vi "acquire-sequence-to-disk-subvi.vi"(0 "Image Size":T7={"H Bin"=1.0, "V Bin"=1.0, "Left"=1.0, "Right"=1024.0, "Top"=1.0, "Bottom"=1024.0} {"V Bin" min=0.0; "H Bin" min=0.0 step=1.0}, 1 "Description Info":string, 2 "Operation":enum16{"Start", "Continue", "Finish"}(ring), 3 "Number of frames to acquire":i32, 5 "Display?":bool, 7 "State In":T1 {"Height" format="%.2f"; "Width" format="%.2f"}, 9 "Frames per acquisition file":u32, 11 "Sequence files handle":T8, 12 "Pressing stop automatically runs finish?":bool=TRUE, 13 "Display Window Title":string="Acquired Image", 14 "Display Window Number":i32) -> (4 "Done?":bool, 6 "State Out":T1 {"Height" format="%.2f"; "Width" format="%.2f"}, 10 "Sequence files handle out":T8, 15 "Error Out":errorcluster)   [LabVIEW 2014]
uses:
  SubVIs/ctt's/Video acquisition state1.ctl
  <vilib>/vision/Image Controls.llb/IMAQ Image.ctl
  Glimpse-master/Glimpse core/Seq file v 1/Offset table.ctl
  Glimpse-master/Glimpse core/Seq file v 1/Offset.ctl
  Glimpse-master/Glimpse core/Seq file v 1/file number.ctl
  Header2 file.ctl
  SubVIs/Initilize Globals.vi
  Stage Control/Stage SubVis/stage-controller-globals.vi
  Shutter Control/Shutter SubVis/Global Shutter Variables - SubVI.vi
  flow-rate-global.vi
  hardware names - global.vi
panel:
  in  "Laser Shutter (to get strings only)":T6(radio)
  out "Frame interval (ms)":i16
  out "TTB element zero":u32
  out "Time of 1st frame":dbl
  out "Frames Acquired":u32(slide) scale=0.0..10000.0
  in  "Stop":bool
  out "Sequence files directory path":path
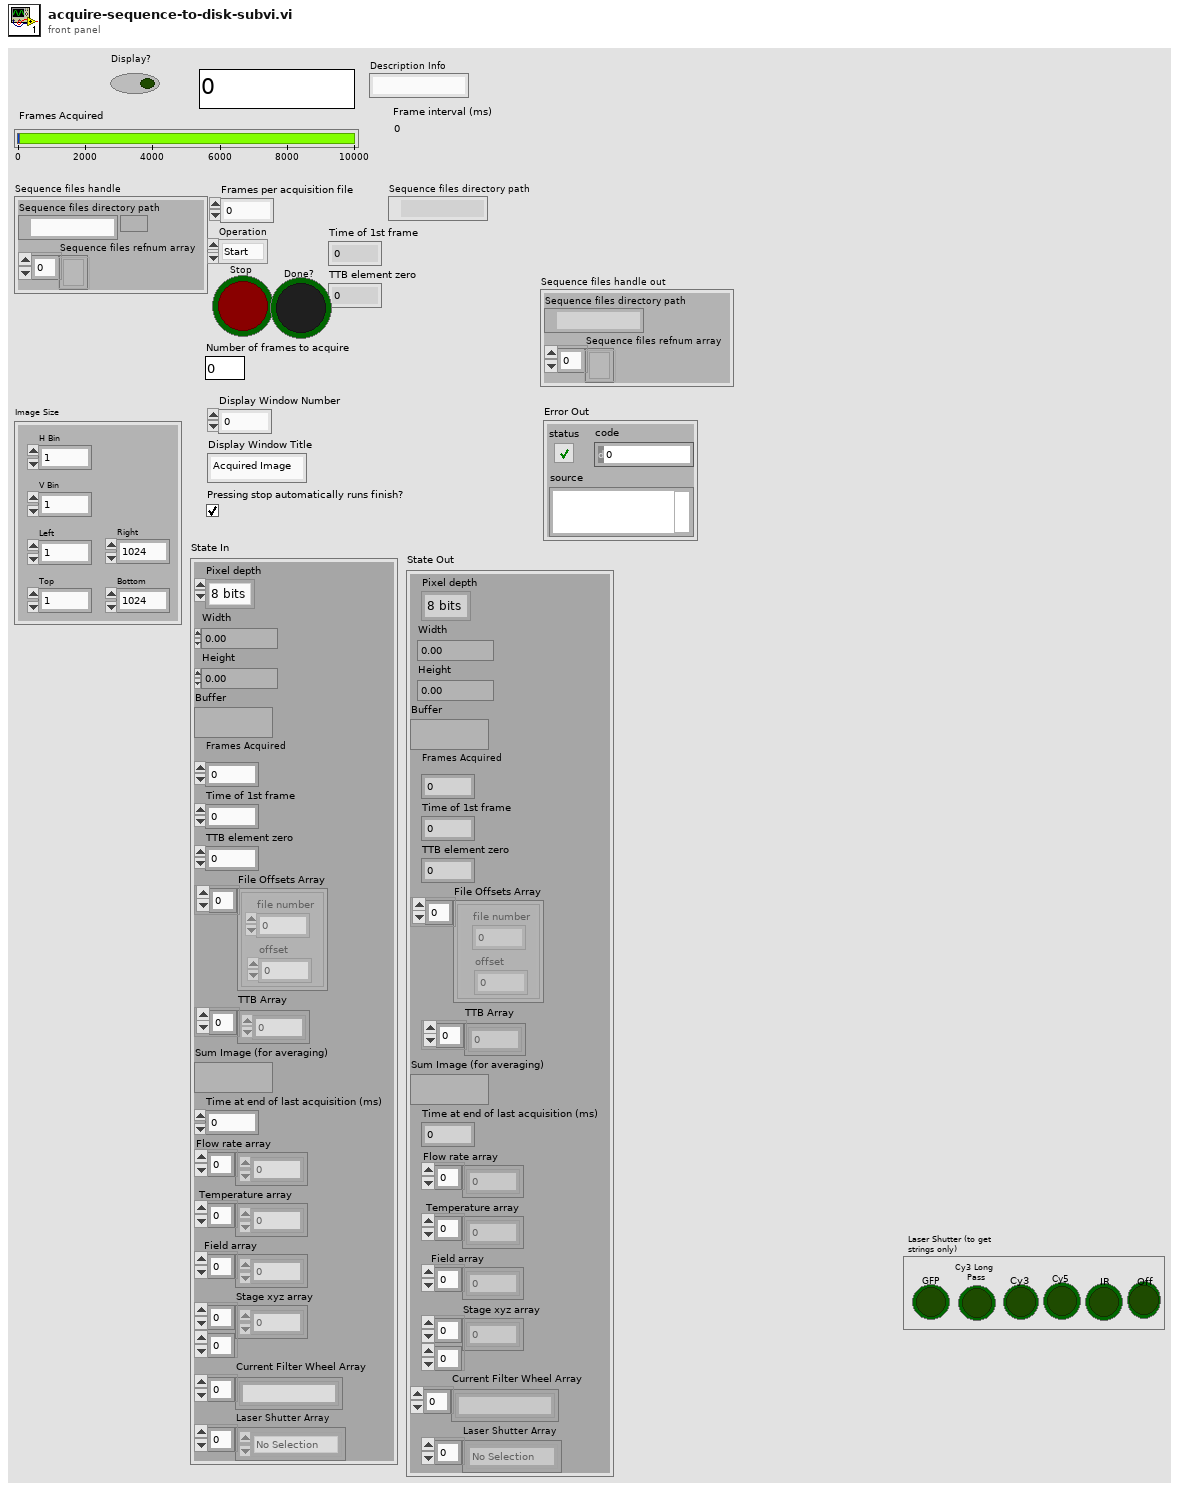
[diagram p1: front panel]
types:
  T1 = typedef "Video acquisition state1.ctl" = cluster{"Pixel depth":enum32{"8 bits", "16 bits", "Float", "Complex", "RGB Chunky", "Compressed"}, "Width":dbl, "Height":dbl, "Buffer":T2, "Frames Acquired":u32, "Time of 1st frame":dbl, "TTB element zero":u32, "File Offsets Array":T3, "TTB Array":u32[], "Sum Image (for averaging)":T2, "Time at end of last acquisition (ms)":u32, "Flow rate array":dbl[], "Temperature array":dbl[], "Field array":u16[], "Stage xyz array":dbl[][], "Current Filter Wheel Array":string[], "Laser Shutter Array":enum32{"No Selection", "GFP", "Cy3 Long \nPass", "Cy3", "Cy5", "Off", "IR"}[]}
  T2 = typedef "IMAQ Image.ctl" = refnum<image>
  T3 = typedef "Offset table.ctl" = cluster{"offset":T4, "file number":T5}[]
  T4 = typedef "Offset.ctl" = i32
  T5 = typedef "file number.ctl" = u8
  T6 = enum32{"No Selection", "GFP", "Cy3 Long \nPass", "Cy3", "Cy5", "Off", "IR"}
  T7 = cluster{"H Bin":dbl, "V Bin":dbl, "Left":dbl, "Right":dbl, "Top":dbl, "Bottom":dbl}
  T8 = cluster{"Sequence files directory path":path, "Sequence files refnum array":refnum<file>[]}
  T9 = enum32{"8 bits", "16 bits", "Float", "Complex", "RGB Chunky", "Compressed"}
  T10 = enum32{"No Selection", "GFP", "Cy3 Long \nPass", "Cy3", "Cy5", "Off", "IR"}[]
  T11 = typedef "Header2 file.ctl" = cluster{"Camera":string, "Microscope":string, "Microscope software version":string, "Flow rate array":dbl[], "Temperature array":dbl[], "Field array":u16[], "Is header2 info present?":bool, "Description Info":string, "Stage xyz array":dbl[][], "Current Filter Wheel Array":string[], "Laser Shutter Array":enum32{"No Selection", "GFP", "Cy3 Long \nPass", "Cy3", "Cy5", "Off", "IR"}[], "Laser Shutter Names":string[]}
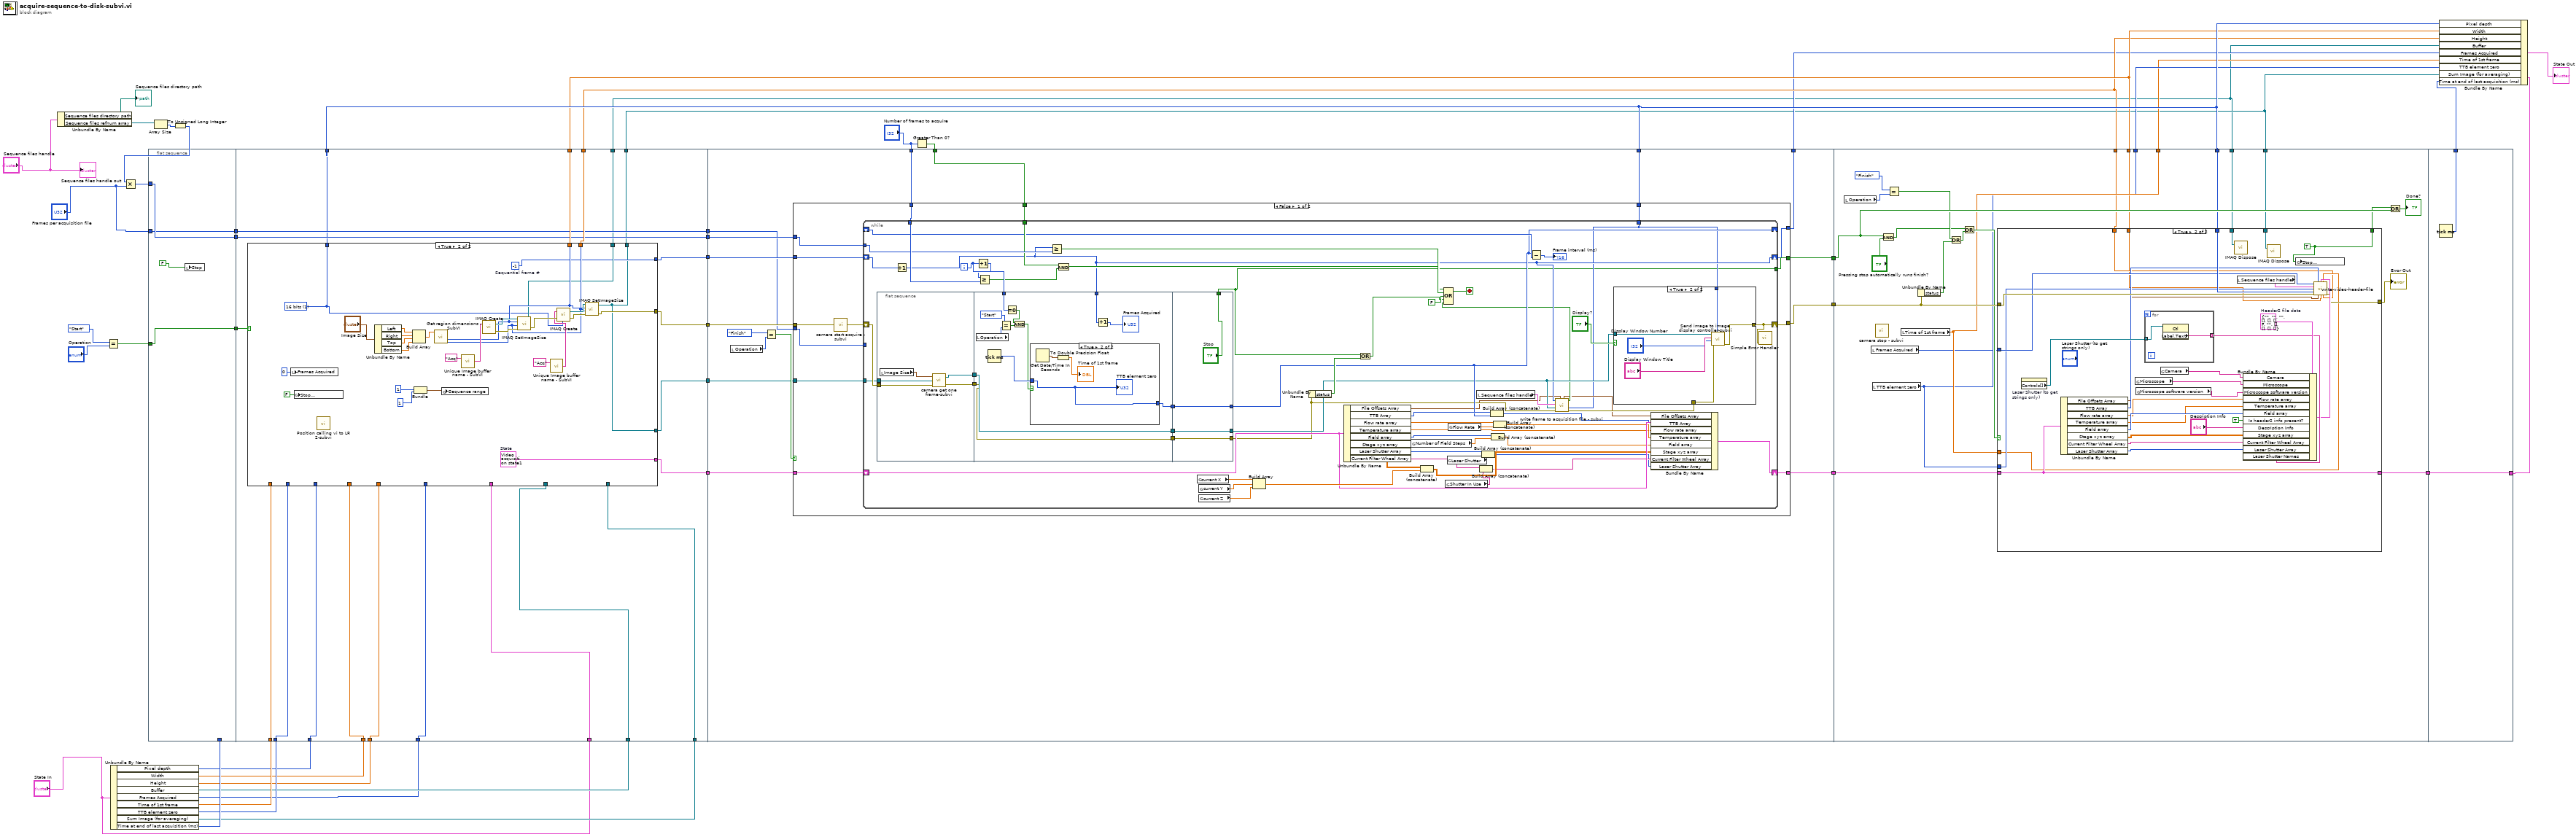
[diagram p0: block diagram]
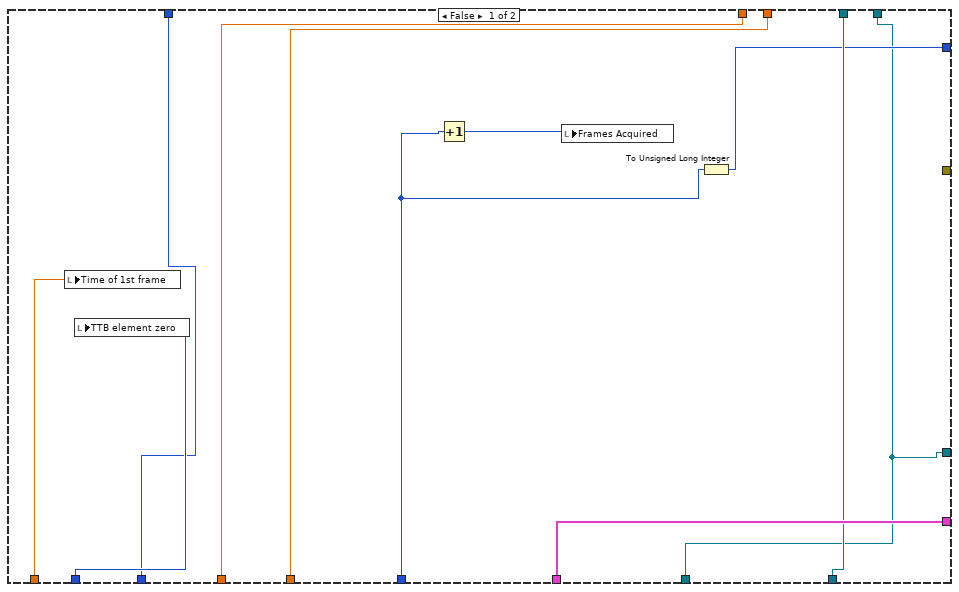
[diagram p2: hidden frame]
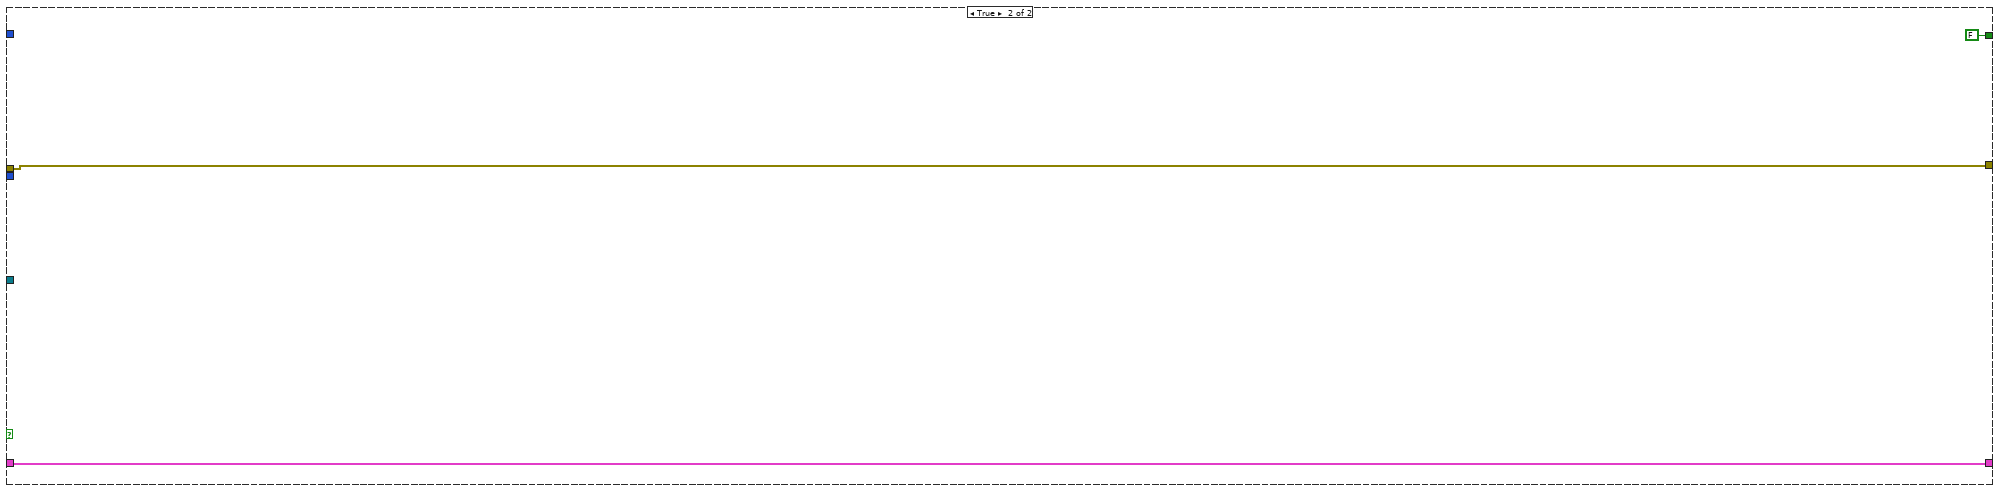
[diagram p5: hidden frame]
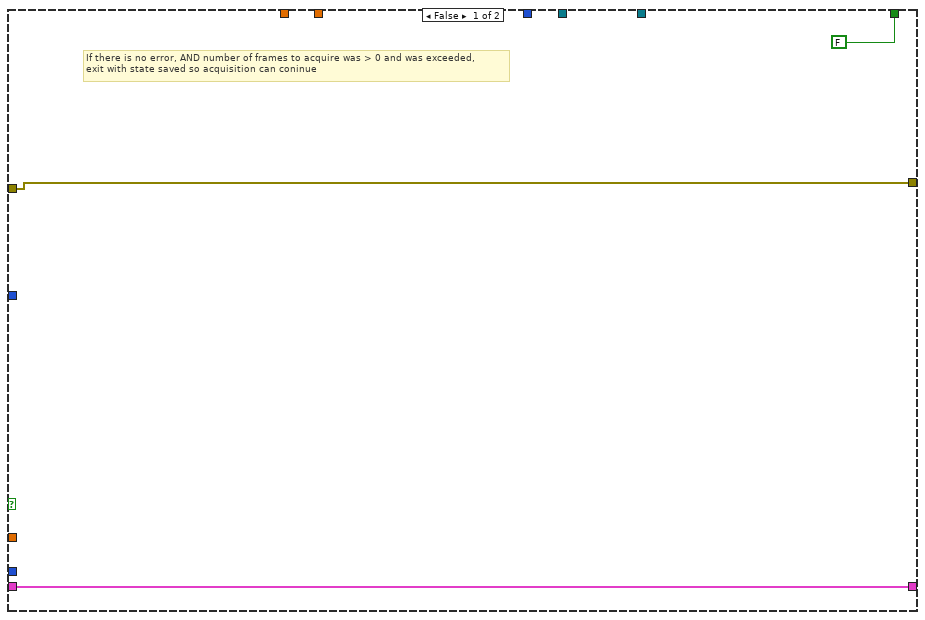
[diagram p6: hidden frame]
diagram:
  n1 = Unbundle By Name("Sequence files handle") -> ("Sequence files directory path"=→"Sequence files directory path":path, "Sequence files refnum array"=w44:refnum<file>[])
  n2 = Equal?(x=enum16{"Start", "Continue", "Finish"}."Start" ("Operation"), y="Operation") -> (x = y?=w38:bool)
  n3 = Unbundle By Name("State In") -> ("Pixel depth"=w29:T9, "Width"=w32:dbl, "Height"=w31:dbl, "Buffer"=w30:T2, "Frames Acquired"=w28:u32, "Time of 1st frame"=w34:dbl, "TTB element zero"=w33:u32, "Sum Image (for averaging)"=w35:T2, "Time at end of last acquisition (ms)"=w36:u32)
  n4 = flat-sequence {
    tunnel: w42 -> [w48]
    tunnel: w38 -> [w50]
    tunnel: [w50] -> w37
    tunnel: w36 -> [_]
    tunnel: [w48] -> w24
    tunnel: "Frames per acquisition file" -> [w47]
    tunnel: [w47] -> w21
    tunnel: w37 -> [w71]
    tunnel: w35 -> [w62]
    tunnel: w34 -> [w70]
    tunnel: w33 -> [w69]
    tunnel: w32 -> [w67]
    tunnel: w31 -> [w66]
    tunnel: "State In" -> [w64]
    tunnel: w30 -> [w63]
    tunnel: w29 -> [w68]
    tunnel: w28 -> [w65]
    tunnel: [w61] -> w7
    tunnel: [w60] -> w6
    tunnel: [w59] -> w27
    tunnel: [w58] -> w26
    tunnel: [w57] -> w25
    tunnel: w24 -> [w57]
    tunnel: [w56] -> w22
    tunnel: w21 -> [w56]
    tunnel: [w55] -> w20
    tunnel: [w54] -> w17
    tunnel: [w53] -> w8
    tunnel: [w52] -> w1
    tunnel: [w51] -> w2
    tunnel: w27 -> [w123]
    tunnel: w26 -> [w122]
    tunnel: w25 -> [w121]
    tunnel: w22 -> [w120]
    tunnel: w20 -> [w119]
    tunnel: w19 -> [w117]
    tunnel: "Number of frames to acquire" -> [w118]
    tunnel: w17 -> [w116]
    tunnel: w8 -> [w115]
    tunnel: [w112] -> w16
    tunnel: [w114] -> w15
    tunnel: [w113] -> w14
    tunnel: [w111] -> w3
    tunnel: w16 -> [w243]
    tunnel: w15 -> [w253]
    tunnel: w14 -> [w252]
    tunnel: [w246] -> w4
    tunnel: [w245] -> w5
    tunnel: w1 -> [w239]
    tunnel: w2 -> [w238]
    tunnel: w6 -> [w237]
    tunnel: w7 -> [w236]
    tunnel: w8 -> [w235]
    tunnel: [w234] -> w12
    tunnel: w12 -> [w293]
    tunnel: [w293] -> w11
    tunnel: [w292] -> w9
    frame #0 {
      n5 = local write "Stop"(FALSE) -> ()
    }
    frame #1 {
      n6 = case shown="True" w71 {
        tunnel: w70 -> [w80 _]
        tunnel: w69 -> [w79 _]
        tunnel: w68 -> [w78 _]
        tunnel: w67 -> [w74 _]
        tunnel: w66 -> [w73 _]
        tunnel: w65 -> [w76 _]
        tunnel: w64 -> [w82 _]
        tunnel: w63 -> [w72 _]
        tunnel: w62 -> [w81 _]
        tunnel: [w78 w85] -> w53
        tunnel: [w82 w95] -> w54
        tunnel: [w74 w89] -> w61
        tunnel: [w73 w88] -> w60
        tunnel: [_ w87] -> w59
        tunnel: [w72 w83] -> w51
        tunnel: [w81 w86] -> w52
        tunnel: [w75 w84] -> w58
        tunnel: [w72 w83] -> w55
        frame False {
          n7 = local write "Time of 1st frame"(w80) -> ()
          n8 = local write "TTB element zero"(w79) -> ()
          n9 = Increment(x=w76) -> (x+1=w77:u32)
          n10 = local write "Frames Acquired"(w77) -> ()
          n11 = To Unsigned Long Integer(number=w76) -> (unsigned 32bit integer=w75:u32)
        }
        frame True {
          w84 = -1  # Sequential frame #
          w85 = u32 1 items=["8 bits", "16 bits", "Float", "Complex", "RGB", "HSL"] ("Image Type")
          w95 = T1 {"Pixel depth"=enum."8 bits", "Width"=0.0, "Height"=0.0, "Buffer"=refnum, "Frames Acquired"=0, "Time of 1st frame"=0.0, "TTB element zero"=0, "File Offsets Array"=[], "TTB Array"=[], "Sum Image (for averaging)"=refnum, "Time at end of last acquisition (ms)"=0, "Flow rate array"=[], "Temperature array"=[], "Field array"=[], "Stage xyz array"=[], "Current Filter Wheel Array"=[], "Laser Shutter Array"=[]}  # State
          n12 = local write "Frames Acquired"(u32 0 ("Frames Acquired")) -> ()
          n13 = global write "Initilize Globals.vi" "Stop \nAcquisition"(FALSE ("Stop \nAcquisition")) -> ()
          n14 = call "Position calling vi to LR 2-subvi.vi"() -> ()  [unwired: 4 in, 2 out]
          n15 = Unbundle By Name("Image Size") -> ("Left"=w109:dbl, "Right"=w108:dbl, "Top"=w107:dbl, "Bottom"=w106:dbl)
          n16 = Build Array(w109, w108, w107, w106) -> (w100:dbl[])
          n17 = Bundle(1, 1) -> (w101:cluster{i32, i32})  [unwired: 1 in]
          n18 = call "Get region dimensions - SubVI.vi"("x1y1x2y2"=w100) -> ("y size"=w88:u16, "x size"=w89:u16)  [unwired: 7 in, 2 out]
          n19 = global write "Initilize Globals.vi" "Sequence range"(w101) -> ()
          n20 = call "Unique Image buffer name - SubVI.vi"("Buffer  base name"="Acq") -> ("Image Name"=w99:string)  [unwired: 1 in]
          n21 = call "IMAQ Create"("Image Name"=w99) -> ("New Image"=w97:T2, "error out"=w96:errorcluster)  [unwired: 4 in]
          n22 = call "IMAQ SetImageSize"("error in (no error)"=w96, "Y Resolution"=w88, "X Resolution"=w89, "Image"=w97) -> ("error out"=w94:errorcluster, "Image Out"=w86:T2)  [unwired: 1 in]
          n23 = call "Unique Image buffer name - SubVI.vi"("Buffer  base name"="Acq") -> ("Image Name"=w92:string)  [unwired: 1 in]
          n24 = call "IMAQ Create"("Image Name"=w92, "Image Type"=w85, "error in (no error)"=w94) -> ("New Image"=w90:T2, "error out"=w91:errorcluster)  [unwired: 2 in]
          n25 = call "IMAQ SetImageSize"("error in (no error)"=w91, "Y Resolution"=w88, "X Resolution"=w89, "Image"=w90) -> ("error out"=w87:errorcluster, "Image Out"=w83:T2)  [unwired: 1 in]
        }
      }
    }
    frame #2 {
      n26 = local read "Operation"() -> (w125:enum16{"Start", "Continue", "Finish"})
      n27 = Equal?(x=enum16{"Start", "Continue", "Finish"}."Finish" ("Operation"), y=w125) -> (x = y?=w124:bool)
      n28 = case shown="False" w124 {
        tunnel: w123 -> [w140 w233]
        tunnel: w122 -> [w138 _]
        tunnel: w121 -> [w137 _]
        tunnel: w120 -> [w136 _]
        tunnel: w119 -> [w135 _]
        tunnel: w118 -> [w134 _]
        tunnel: w117 -> [w133 _]
        tunnel: w116 -> [w132 w231]
        tunnel: [w131 w233] -> w113
        tunnel: w115 -> [w130 _]
        tunnel: [w129 w231] -> w112
        tunnel: [w128 FALSE ("Stop")] -> w114
        tunnel: [w127 _] -> w111
        frame False {
          n29 = call "camera start acquire - subvi.vi"("error in"=w140) -> ("error out"=w139:errorcluster)
          n30 = while {
            shift-right: [w170] -> w131
            shift-left: w139 -> [w198]
            shift-right: [w147] -> w127
            shift-left: w138 -> [w188]
            tunnel: w137 -> [w187]
            tunnel: w136 -> [_]
            tunnel: w135 -> [w197]
            tunnel: w134 -> [w189]
            tunnel: w133 -> [w185]
            shift-right: [w163] -> w129
            shift-left: w132 -> [w164]
            shift-right: [w152] -> _
            shift-left: _ -> [w173]
            tunnel: w130 -> [w142]
            tunnel: [w141] -> w128
            i -> [w191]
            stop <- w184 stop-if-true
            n31 = flat-sequence {
              tunnel: w198 -> [w209]
              tunnel: w197 -> [w208]
              tunnel: [w207] -> w196
              tunnel: [w206] -> w195
              tunnel: w196 -> [w214]
              tunnel: w195 -> [w215]
              tunnel: [w215] -> w194
              tunnel: [w214] -> w193
              tunnel: [w213] -> w192
              tunnel: w191 -> [w212]
              tunnel: w147 -> [w211]
              tunnel: [w229] -> w148
              tunnel: [w230] -> w149
              tunnel: w194 -> [w230]
              tunnel: w193 -> [w229]
              tunnel: [w228] -> w152
              tunnel: w192 -> [w228]
              tunnel: ["Stop"] -> w141
              frame #0 {
                n32 = local read "Image Size"() -> (w210:T7)
                n33 = call "camera get one frame-subvi.vi"("error in"=w209, "New Image"=w208, "Image Size"=w210) -> ("error out"=w207:errorcluster, "Image Out"=w206:T2)
              }
              frame #1 {
                n34 = local read "Operation"() -> (w217:enum16{"Start", "Continue", "Finish"})
                n35 = Tick Count (ms)() -> (millisecond timer value=w222:u32)
                n36 = Equal?(x=enum16{"Start", "Continue", "Finish"}."Start" ("Operation"), y=w217) -> (x = y?=w219:bool)
                n37 = Equal To 0?(x=w212) -> (x = 0?=w216:bool)
                n38 = And(x=w216, y=w219) -> (x .and. y?=w220:bool)
                n39 = case shown="True" w220 {
                  tunnel: w222 -> [w223 w226]
                  tunnel: [w223 w226] -> w213
                  frame False {
                  }
                  frame True {
                    n40 = Get Date/Time In Seconds() -> (seconds since 1Jan1904=w225:timestamp)
                    n41 = To Double Precision Float(number=w225) -> (double precision float=→"Time of 1st frame":dbl)
                    "TTB element zero" <- w226
                  }
                }
                n42 = Increment(x=w211) -> (x+1=→"Frames Acquired":u32)
              }
              frame #2 {
              }
            }
            n43 = Increment(x=w188) -> (x+1=w147:u32)
            n44 = Increment(x=w191) -> (x+1=w190:i32)
            n45 = Greater Or Equal?(x=w190, y=w189) -> (x >= y?=w186:bool)
            n46 = Greater Or Equal?(x=w147, y=w187) -> (x >= y?=w182:bool)
            n47 = And(x=w185, y=w186) -> (x .and. y?=w181:bool)
            n48 = global read "stage-controller-globals.vi" "current X"() -> (w178:dbl)
            n49 = global read "stage-controller-globals.vi" "current Y"() -> (w177:dbl)
            n50 = global read "stage-controller-globals.vi" "current Z"() -> (w176:dbl)
            n51 = Build Array(w178, w177, w176) -> (w175:dbl[])
            n52 = Unbundle By Name(w148) -> ("status"=w179:bool)
            n53 = Unbundle By Name(w164) -> ("File Offsets Array"=w144:T3, "TTB Array"=w169:u32[], "Flow rate array"=w167:dbl[], "Temperature array"=w161:dbl[], "Field array"=w168:u16[], "Stage xyz array"=w174:dbl[][], "Laser Shutter Array"=w166:T10, "Current Filter Wheel Array"=w165:string[])
            n54 = Or(x=w141, y=w179) -> (x .or. y?=w180:bool)
            n55 = global read "stage-controller-globals.vi" "Number of Field Steps"() -> (w156:dbl)
            n56 = Build Array (concatenate)(w174, w175) -> (w162:dbl[][])
            n57 = global read "Global Shutter Variables - SubVI.vi" "Shutter In Use"() -> (w160:string)
            n58 = global read "Global Shutter Variables - SubVI.vi" "Laser Shutter"() -> (w158:T6)
            n59 = global read "flow-rate-global.vi" "Flow Rate"() -> (w154:dbl)
            n60 = local read "Sequence files handle"() -> (w150:T8)
            n61 = Build Array (concatenate)(w165, w160) -> (w159:string[])
            n62 = Build Array (concatenate)(w166, w158) -> (w157:T10)
            n63 = Build Array (concatenate)(w169, w152) -> (w151:u32[])
            n64 = Build Array (concatenate)(w168, w156) -> (w155:dbl[])
            n65 = Build Array (concatenate)(w167, w154) -> (w153:dbl[])
            n66 = Subtract(x=w152, y=w173) -> (x-y=→"Frame interval (ms)":u32)
            n67 = call "write frame to acquisition file - subvi.vi"("Pixel depth"=w142, "Offset table in"=w144, "Error In"=w148, "Image In"=w149, "Sequence files handle"=w150, "Last frame number written in"=w147) -> ("Error Out"=w145:errorcluster, "Stop"=w146:bool, "Offset table out"=w143:cluster{"offset":i32, "file number":u8}[])  [unwired: 2 in, 1 out]
            n68 = Compound Arithmetic op=OR(w181, w182, FALSE, w180, w146) -> (w184:bool)
            n69 = case shown="True" "Display?" {
              tunnel: [w199 w205] -> w170
              tunnel: w145 -> [w199 w202]
              tunnel: w149 -> [_ w201]
              tunnel: w142 -> [_ w200]
              frame False {
              }
              frame True {
                n70 = call "Send image to image display controller-subvi.vi"("Image"=w201, "Window Title"="Display Window Title", "Window Number"="Display Window Number", "error in"=w202, "Image Type"=w200) -> ("error out"=w205:errorcluster)  [unwired: 4 in, 1 out]
              }
            }
            n71 = Bundle By Name(cluster=w164, "File Offsets Array"=w143, "TTB Array"=w151, "Flow rate array"=w153, "Temperature array"=w161, "Field array"=w155, "Stage xyz array"=w162, "Current Filter Wheel Array"=w159, "Laser Shutter Array"=w157) -> (w163:T1)
            n72 = call <vilib>:"Simple Error Handler.vi"("error in (no error)"=w170) -> ()  [unwired: 4 in, 5 out]
          }
        }
        frame True {
        }
      }
    }
    frame #3 {
      n73 = local read "Operation"() -> (w256:enum16{"Start", "Continue", "Finish"})
      n74 = local read "Frames Acquired"() -> (w244:u32)
      n75 = local read "TTB element zero"() -> (w245:u32)
      n76 = call "camera stop - subvi.vi"() -> ()  [unwired: 1 in]
      n77 = And(x=w253, y="Pressing stop automatically runs finish?") -> (x .and. y?=w249:bool)
      n78 = Equal?(x=enum16{"Start", "Continue", "Finish"}."Finish" ("Operation"), y=w256) -> (x = y?=w250:bool)
      n79 = local read "Time of 1st frame"() -> (w246:dbl)
      n80 = Unbundle By Name(w252) -> ("status"=w251:bool)
      n81 = Or(x=w250, y=w251) -> (x .or. y?=w248:bool)
      n82 = Or(x=w249, y=w248) -> (x .or. y?=w247:bool)
      n83 = case shown="True" w247 {
        tunnel: w252 -> [w258 w269]
        tunnel: w246 -> [_ w262]
        tunnel: w245 -> [_ w263]
        tunnel: w244 -> [_ w266]
        tunnel: w243 -> [w259 w288]
        tunnel: [w259 w288] -> w234
        tunnel: [w258 w270] -> w242
        tunnel: [FALSE w289] -> w241
        tunnel: w239 -> [_ w275]
        tunnel: w238 -> [_ w274]
        tunnel: w237 -> [_ w261]
        tunnel: w236 -> [_ w260]
        tunnel: w235 -> [_ w268]
        frame False {
          # "If there is no error, AND number of frames to acquire was > 0 and was exceeded,\nexit with state saved so acquisition can coninue"
        }
        frame True {
          w287 = T11 {"Camera"="", "Microscope"="", "Microscope software version"="", "Flow rate array"=[], "Temperature array"=[], "Field array"=[], "Is header2 info present?"=FALSE, "Description Info"="", "Stage xyz array"=[], "Current Filter Wheel Array"=[], "Laser Shutter Array"=[], "Laser Shutter Names"=[]}  # Header2 file data
          w289 = TRUE
          n84 = property on="Laser Shutter (to get strings only)" class="RadioBtnsControl (strict)"() -> ("Controls[]"=w273:refnum<vi>[])  [unwired: 2 in, 2 out]
          n85 = Unbundle By Name(w288) -> ("File Offsets Array"=w264:T3, "TTB Array"=w265:u32[], "Flow rate array"=w281:dbl[], "Temperature array"=w282:dbl[], "Field array"=w286:u16[], "Stage xyz array"=w283:dbl[][], "Current Filter Wheel Array"=w284:string[], "Laser Shutter Array"=w285:T10)
          n86 = global read "hardware names - global.vi" "Microscope"() -> (w277:string)
          n87 = global read "hardware names - global.vi" "Microscope software version"() -> (w276:string)
          n88 = for {
            tunnel: w273 -> [w291] mode=indexing
            tunnel: [w290] -> w272 mode=indexing
            n89 = property class="Ctl"(reference=w291) -> ("Label.Text"=w290:string)  [unwired: 1 in, 2 out]
          }
          n90 = global read "hardware names - global.vi" "Camera"() -> (w278:string)
          n91 = call "IMAQ Dispose"("Image"=w275) -> ()  [unwired: 2 in, 4 out]
          n92 = local read "Sequence files handle"() -> (w267:T8)
          n93 = Bundle By Name(cluster=w287, "Camera"=w278, "Microscope"=w277, "Microscope software version"=w276, "Flow rate array"=w281, "Temperature array"=w282, "Field array"=w286, "Is header2 info present?"=TRUE, "Description Info"="Description Info", "Stage xyz array"=w283, "Current Filter Wheel Array"=w284, "Laser Shutter Array"=w285, "Laser Shutter Names"=w272) -> (w271:T11)
          n94 = call "IMAQ Dispose"("Image"=w274) -> ()  [unwired: 2 in, 4 out]
          n95 = global write "Initilize Globals.vi" "Stop \nAcquisition"(w289) -> ()
          n96 = call "write-video-header-file.vi"("Frames Acquired"=w266, "TTB Array (ms)"=w265, "Header2 file data"=w271, "time of 1st frame, \nsec"=w262, "Sequence files handle"=w267, "Element 0 of TTB"=w263, "Pixel depth\n(0=8 bit; 1= 16 bit)"=w268, "Error In"=w269, "File Offsets Array"=w264, "Region width"=w260, "Region height"=w261) -> ("Error Out"=w270:errorcluster)  [unwired: 4 in]
        }
      }
      "Error Out" <- w242
      n97 = Or(x=w241, y=w253) -> (x .or. y?=→"Done?":bool)
    }
    frame #4 {
      n98 = Tick Count (ms)() -> (millisecond timer value=w292:u32)
    }
  }
  n99 = Array Size(array=w44) -> (size(s)=w43:i32)
  n100 = To Unsigned Long Integer(number=w43) -> (unsigned 32bit integer=w41:u32)
  n101 = Multiply(x=w41, y="Frames per acquisition file") -> (x*y=w42:u32)
  n102 = Greater Than 0?(x="Number of frames to acquire") -> (x > 0?=w19:bool)
  n103 = Bundle By Name(cluster=w11, "Pixel depth"=w8, "Width"=w7, "Height"=w6, "Buffer"=w1, "Frames Acquired"=w3, "Time of 1st frame"=w4, "TTB element zero"=w5, "Sum Image (for averaging)"=w2, "Time at end of last acquisition (ms)"=w9) -> (→"State Out":T1)
  "Sequence files handle out" <- "Sequence files handle"
